vi "array-icicle-manage.vi"(0 "icicle array IN":T2[](array[typedef]), 1 "action":T1, 5 "string array IN":string[](array[string]), 11 "string in":string) -> (4 "icicle array OUT":T2[](array[typedef]), 6 "string array OUT":string[](array[string]), 8 "number array out":dbl[](array[numeric]), 10 "number out":dbl, 15 "string out":string)   [LabVIEW 2020]
uses:
  icicle.ctl
  array-icicle-manage-action.ctl
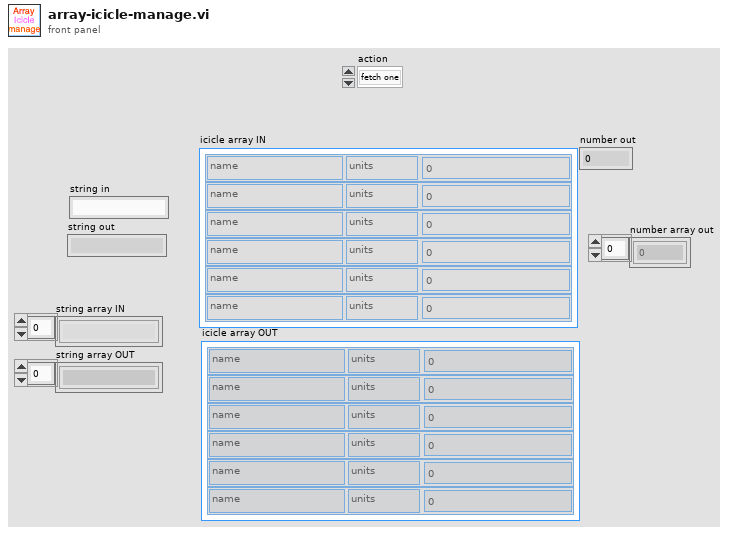
[diagram p1: front panel]
types:
  T1 = typedef "array-icicle-manage-action.ctl" = enum16{"fetch one", "fetch a few"}
  T2 = typedef "icicle.ctl" = cluster{"name":string, "units":string, "data":dbl}
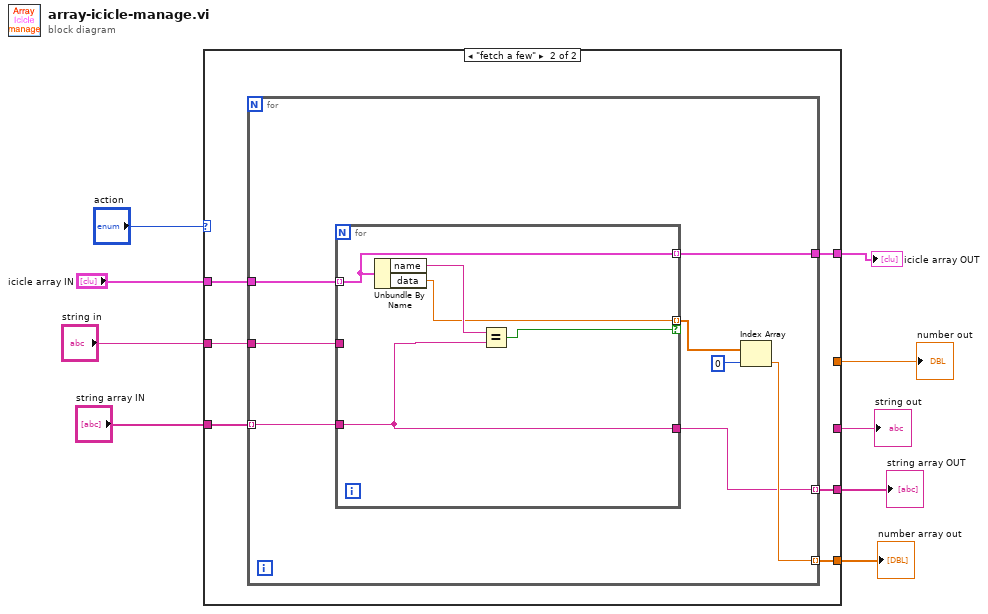
[diagram p0: block diagram]
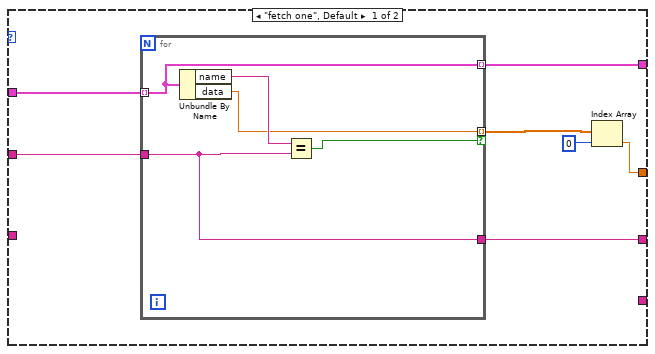
[diagram p2: hidden frame]
diagram:
  n1 = case shown="\"fetch a few\"" "action" {
    tunnel: "icicle array IN" -> [w16 w27]
    tunnel: "string in" -> [w15 w26]
    tunnel: [w14 w25] -> w6
    tunnel: [w13 _] -> w5
    tunnel: [w10 _] -> w4
    tunnel: "string array IN" -> [_ w24]
    tunnel: [_ w23] -> w2
    tunnel: [_ w22] -> w1
    frame "fetch one", Default {
      n2 = for {
        tunnel: w16 -> [w18] mode=indexing
        tunnel: w15 -> [w17]
        tunnel: [w20] -> w11 mode=indexing if=w19
        tunnel: [w18] -> w14 mode=indexing
        tunnel: [w17] -> w13
        n3 = Unbundle By Name(w18) -> ("name"=w21:string, "data"=w20:dbl)
        n4 = Equal?(x=w21, y=w17) -> (x = y?=w19:bool)
      }
      n5 = Index Array(array=w11, index=0) -> (element=w10:dbl)
    }
    frame "fetch a few" {
      n6 = for {
        tunnel: w27 -> [w35]
        tunnel: [w33] -> w25
        tunnel: w26 -> [w34]
        tunnel: w24 -> [w30] mode=indexing
        tunnel: [w29] -> w23 mode=indexing
        tunnel: [w28] -> w22 mode=indexing
        n7 = for {
          tunnel: w35 -> [w37] mode=indexing
          tunnel: w34 -> [_]
          tunnel: [w39] -> w32 mode=indexing if=w38
          tunnel: [w37] -> w33 mode=indexing
          tunnel: [w36] -> w28
          tunnel: w30 -> [w36]
          n8 = Unbundle By Name(w37) -> ("name"=w40:string, "data"=w39:dbl)
          n9 = Equal?(x=w40, y=w36) -> (x = y?=w38:bool)
        }
        n10 = Index Array(array=w32, index=0) -> (element=w29:dbl)
      }
    }
  }
  "icicle array OUT" <- w6
  "string out" <- w5
  "number out" <- w4
  "string array OUT" <- w1
  "number array out" <- w2
